vi "Check out.vi"(8 "error in (no error)":errorcluster, 11 "reference Class in":refnum<class "Reference Class.lvclass">) -> (0 "error out":errorcluster, 2 "data":refnum<class "Simple Class.lvclass">, 3 "reference Class out":refnum<class "Reference Class.lvclass">)   [LabVIEW 2023, in "Reference Class.lvclass"]
doc: "Check out the object. Any other attempts to check out the object will wait for the object to be checked back in."
uses:
  Reference Class.lvclass
  SimpleClass/Simple Class.lvclass
  Reference Class.lvclass/Reference Class.ctl
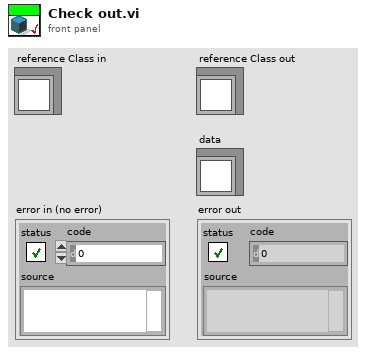
[diagram p1: front panel]
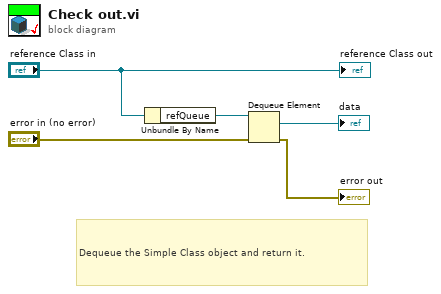
[diagram p0: block diagram]
diagram:
  # "Dequeue the Simple Class object and return it."
  n1 = Unbundle By Name("reference Class in") -> ("refQueue"=w4:refnum<queue>)
  n2 = Dequeue Element(queue=w4, error in (no error)="error in (no error)") -> (element=→"data":refnum<class "Simple Class.lvclass">, error out=→"error out":errorcluster)  [unwired: 1 in, 2 out]
  "reference Class out" <- "reference Class in"
